vi "Handle Response.vi"(8 "error in (no error)":errorcluster, 9 "Body":string, 10 "Headers":string, 11 "Gmail in":refnum<class "Gmail.lvclass">) -> (0 "error out":errorcluster, 3 "Gmail out":refnum<class "Gmail.lvclass">, 5 "Refresh?":bool)   [LabVIEW 2020, in "Gmail API.lvlib" / "Gmail.lvclass"]
uses:
  Gmail.lvclass
  Gmail.lvclass/Gmail.ctl
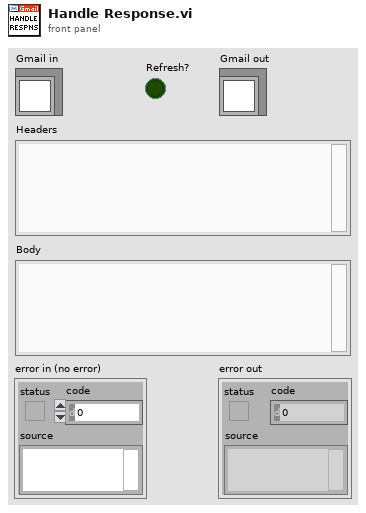
[diagram p1: front panel]
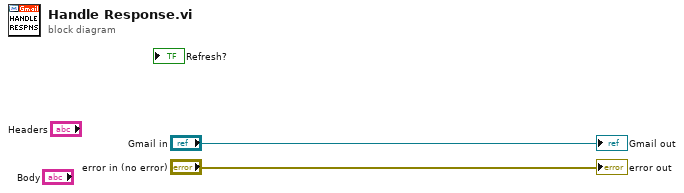
[diagram p0: block diagram]
diagram:
  "error out" <- "error in (no error)"
  "Gmail out" <- "Gmail in"
